vi "stage_get_status.vi"(8 "error in (no error)":errorcluster, 10 "Stage Name":string, 11 "newport_xps in":refnum<class "newport_xps.lvclass">) -> (0 "error out":errorcluster, 2 "Status":string, 3 "newport_xps out":refnum<class "newport_xps.lvclass">)   [LabVIEW 2015, in "newport_xps.lvclass"]
uses:
  newport_xps.lvclass
  newport_xps.lvclass/newport_xps.ctl
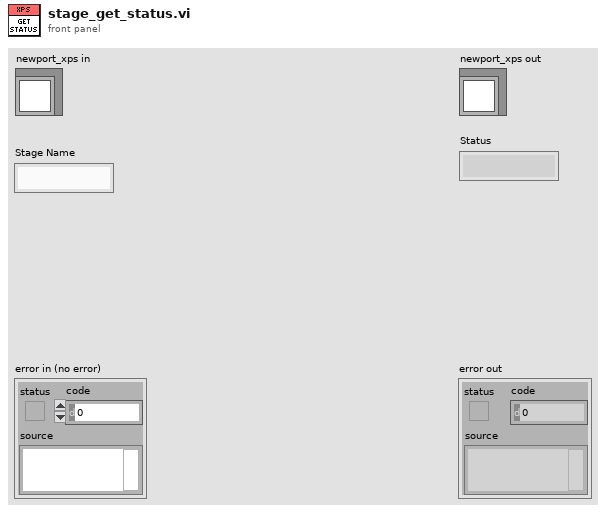
[diagram p1: front panel]
types:
  T1 = cluster{"connection TCP":refnum<k5>, "LogTo File":bool, "Log File refnum":refnum<file>, "no error if error log":bool}
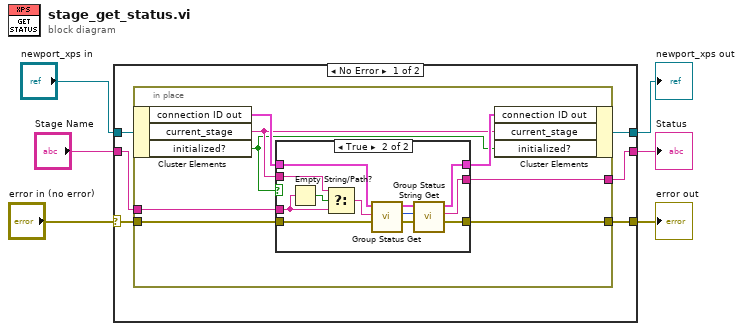
[diagram p0: block diagram]
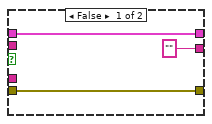
[diagram p2: hidden frame]
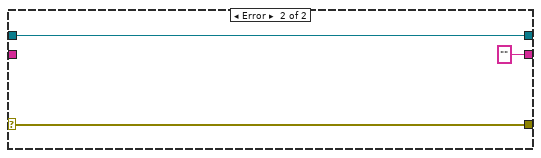
[diagram p3: hidden frame]
diagram:
  n1 = case shown="No Error" "error in (no error)" {
    selector: "error in (no error)" -> [w9 w37]
    tunnel: "newport_xps in" -> [w12 w38]
    tunnel: [w11 "" ("Group Status String")] -> w4
    tunnel: "Stage Name" -> [w10 _]
    tunnel: [w8 w37] -> w2
    tunnel: [w7 w38] -> w1
    frame No Error {
      n2 = in-place {
        in-place-border: [w19] -> w11
        in-place-border: w10 -> [w18]
        in-place-border: w9 -> [w17]
        in-place-border: [w16] -> w8
        n3 = in-place-cluster #1(w12) -> ("connection ID out"=w20:T1, "current_stage"=w14:string, "initialized?"=w13:bool)
        n4 = case shown="True" w13 {
          tunnel: w20 -> [w21 w35]
          tunnel: ["" ("Group Status String") w32] -> w19
          tunnel: w18 -> [_ w30]
          tunnel: w17 -> [w23 w28]
          tunnel: [w23 w27] -> w16
          tunnel: [w21 w26] -> w15
          tunnel: w14 -> [_ w25]
          frame False {
          }
          frame True {
            n5 = Empty String/Path?(string/path=w30) -> (empty?=w31:bool)
            n6 = Select(t=w25, s=w31, f=w30) -> (s? t:f=w29:string)
            n7 = call "Group Status Get.vi"("XPS error in (no error)"=w28, "Group Name (250 c max)"=w29, "connection ID in"=w35) -> ("XPS error out"=w24:errorcluster, "Status"=w33:i32, "connection ID out"=w34:T1)  [unwired: 5 in, 1 out]
            n8 = call "Group Status String Get.vi"("XPS error in (no error)"=w24, "Status #"=w33, "connection ID in"=w34) -> ("XPS error out"=w27:errorcluster, "Group Status String"=w32:string, "connection ID out"=w26:T1)  [unwired: 5 in, 1 out]
          }
        }
        n9 = in-place-cluster #1("connection ID out"=w15, "current_stage"=w14, "initialized?"=w13) -> (w7:refnum<class "newport_xps.lvclass">)
      }
    }
    frame Error {
    }
  }
  "error out" <- w2
  "newport_xps out" <- w1
  "Status" <- w4
